vi "Acq.vi"(8 "error in (no error)":errorcluster, 11 "Stage_MadCityLab in":refnum<class "Stage_MadCityLab.lvclass">) -> (0 "error out":errorcluster, 3 "Stage_MadCityLab out":refnum<class "Stage_MadCityLab.lvclass">)   [LabVIEW 2020, in "Stage_MadCityLab.lvlib" / "Stage_MadCityLab.lvclass"]
uses:
  Stage_MadCityLab.lvclass
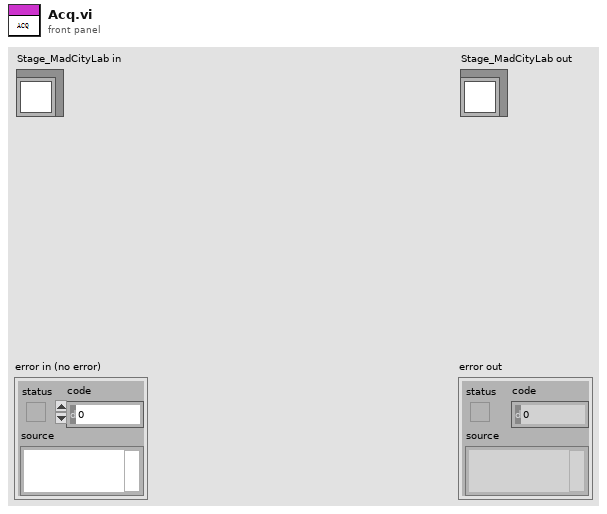
[diagram p1: front panel]
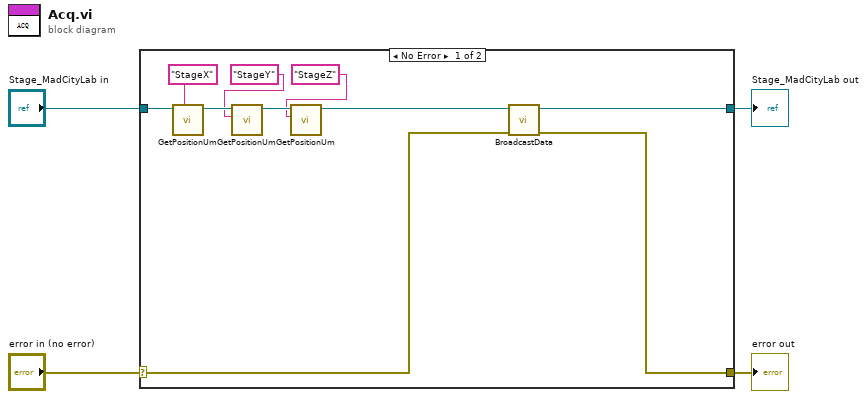
[diagram p0: block diagram]
diagram:
  n1 = case shown="No Error" "error in (no error)" {
    selector: "error in (no error)" -> [w6 w16]
    tunnel: [w5 w16] -> w3
    tunnel: [w7 w15] -> w1
    tunnel: "Stage_MadCityLab in" -> [w14 w15]
    frame No Error {
      n2 = call-dynamic "GetPositionUm.vi"("Stage Label"="StageX", "Stage_MadCityLab in"=w14) -> ("Stage_MadCityLab out"=w13:refnum<class "Stage_MadCityLab.lvclass">)  [unwired: 7 in, 2 out]
      n3 = call-dynamic "GetPositionUm.vi"("Stage Label"="StageY", "Stage_MadCityLab in"=w13) -> ("Stage_MadCityLab out"=w12:refnum<class "Stage_MadCityLab.lvclass">)  [unwired: 7 in, 2 out]
      n4 = call-dynamic "GetPositionUm.vi"("Stage Label"="StageZ", "Stage_MadCityLab in"=w12) -> ("Stage_MadCityLab out"=w11:refnum<class "Stage_MadCityLab.lvclass">)  [unwired: 7 in, 2 out]
      n5 = call-dynamic "BroadcastData.vi"("error in (no error)"=w6, "Device in"=w11) -> ("error out"=w5:errorcluster, "Device out"=w7:refnum<class "Stage_MadCityLab.lvclass">)  [unwired: 8 in]
    }
    frame Error {
    }
  }
  "error out" <- w3
  "Stage_MadCityLab out" <- w1
